vi "Test Sequence Constructor.vi"() -> ()   [LabVIEW 2014]
panel:
  in  "Sequence 2":string(tree)
  out "Steps":string[](array[string])
  out "Values":string[](array[string])
  in  "add":bool
  in  "Steps":string(tree)
  in  "Sequence":string(tree)
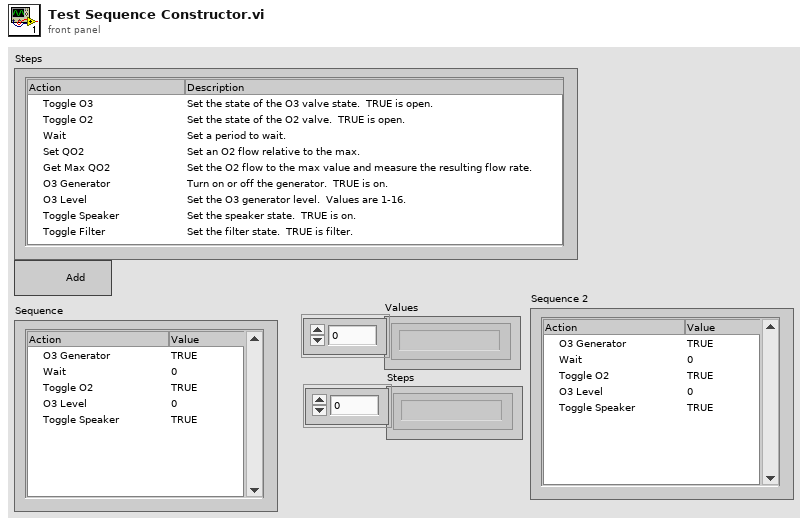
[diagram p1: front panel]
types:
  T1 = typedef "eventvkey.ctl" = enum16{"ASCII", "Enter", "Return", "Shift", "Ctrl", "Alt", "Cmd", "Opt", "Caps", "NumLock", "Clear", "Break", "Up", "Down", "Left", "Right", "Insert", "Delete", "Home", "End", "PageUp", "PageDown", "Escape", "Help", "Pause", "ScrollLock", "F1", "F2", "F3", "F4", "F5", "F6", "F7", "F8", "F9", "F10", "F11", "F12", "F13", "F14", "F15", "F16", "F17", "F18", "F19", "F20", "F21", "F22", "F23", "F24", "Play", "VolumeUp", "VolumeDown", "Mute", "Two Byte Char"}
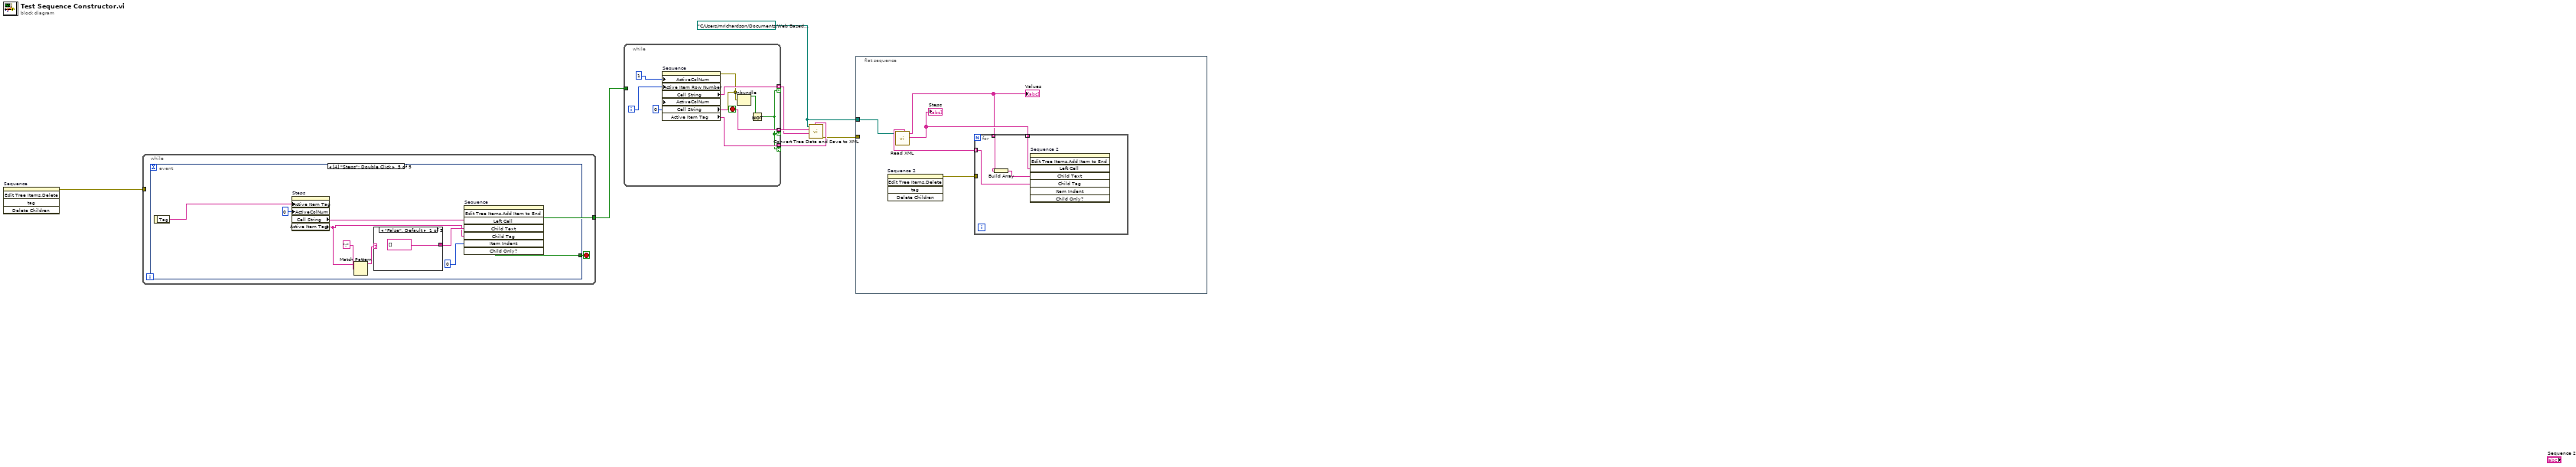
[diagram p0: block diagram]
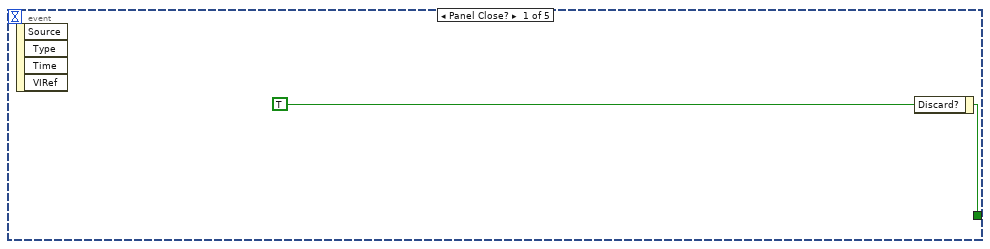
[diagram p2: hidden frame]
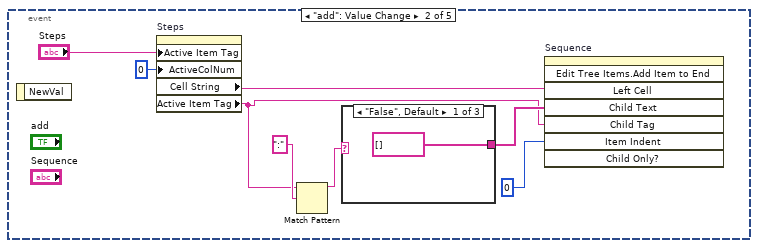
[diagram p3: hidden frame]
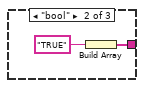
[diagram p4: hidden frame]
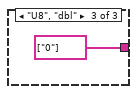
[diagram p5: hidden frame]
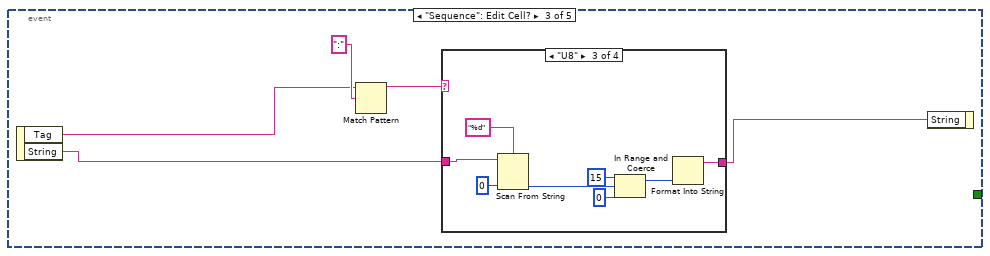
[diagram p6: hidden frame]
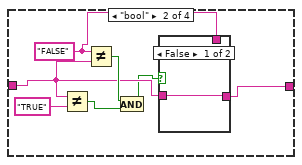
[diagram p8: hidden frame]
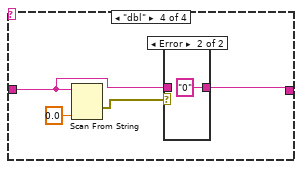
[diagram p10: hidden frame]
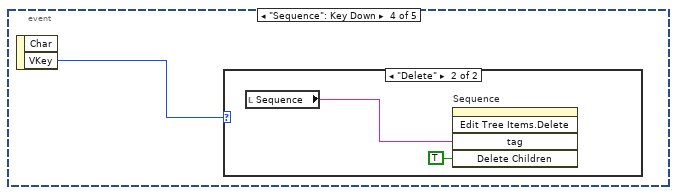
[diagram p12: hidden frame]
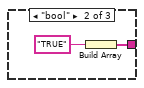
[diagram p14: hidden frame]
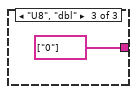
[diagram p15: hidden frame]
diagram:
  w1 = path "C:/Users/mrichardson/Documents/Web Based Version Control SW/Instruments/cPAS/Test/test.xml" ("file")
  n1 = invoke on="Sequence" class="Tree (strict)" method="Edit Tree Items.Delete"() -> (error out=w7:errorcluster)  [unwired: 5 in, 4 out]
  n2 = while {
    tunnel: w7 -> [_]
    tunnel: [w8] -> w6
    stop <- w8 stop-if-true
    n3 = event shown="[4] \"Steps\": Double Click" {
      selector: _ -> [_ _ _ _ _]
      dyn-events: _ -> [_ _ _ _ _]
      timeout: _ -> [_ _ _ _ _]
      tunnel: [w9 _ _ _ _] -> w8
      event Panel Close? {
        w9 = TRUE ("Discard?")
        n4 = event-data() -> ()  [unwired: 1 in, 4 out]
        n5 = event-data("Discard?"=w9) -> ()  [unwired: 1 in, 1 out]
      }
      event "add": Value Change {
        n6 = event-data() -> ()  [unwired: 1 in, 1 out]
        n7 = property on="Steps" class="Tree (strict)"("Active Item Tag"="Steps", "ActiveColNum"=0 ("Active Cell:Active Column Number")) -> ("Cell String"=w15:string, "Active Item Tag"=w10:string)  [unwired: 2 in, 2 out]
        n8 = Match Pattern(string=w10, regular expression=":" ("search string/char (-)")) -> (before substring=w11:string)  [unwired: 1 in, 3 out]
        n9 = case shown="\"False\", Default" w11 {
          tunnel: [string[] [] w19 string[] ["0"]] -> w13
          frame "False", Default {
          }
          frame "bool" {
            n10 = Build Array("TRUE") -> (w19:string[])
          }
          frame "U8", "dbl" {
          }
        }
        n11 = invoke on="Sequence" class="Tree (strict)" method="Edit Tree Items.Add Item to End"("Left Cell"=w15, "Child Text"=w13, "Child Tag"=w10, "Item Indent"=0 ("New Item Indentation")) -> ()  [unwired: 4 in, 8 out]
      }
      event "Sequence": Edit Cell? {
        n12 = event-data() -> ("Tag"=w22:string, "String"=w24:string)  [unwired: 1 in]
        n13 = Match Pattern(string=w22, regular expression=":" ("search string/char (-)")) -> (before substring=w25:string)  [unwired: 1 in, 3 out]
        n14 = case shown="\"U8\"" w25 {
          tunnel: w24 -> [w27 w31 w44 w46]
          tunnel: [w27 w28 w37 w45] -> w23
          frame "False", Default {
          }
          frame "bool" {
            w29 = "FALSE" ("x")
            n15 = Not Equal?(x=w31, y="TRUE") -> (x != y?=w33:bool)
            n16 = Not Equal?(x=w29, y=w31) -> (x != y?=w32:bool)
            n17 = And(x=w32, y=w33) -> (x .and. y?=w30:bool)
            n18 = case shown="False" w30 {
              tunnel: w31 -> [w35 _]
              tunnel: [w35 w36] -> w28
              tunnel: w29 -> [_ w36]
              frame False {
              }
              frame True {
              }
            }
          }
          frame "U8" {
            n19 = Scan From String(format string="%d", input string=w44, default 1=u8 0 ("default value 1")) -> (output 1=w41:u8)  [unwired: 2 in, 3 out]
            n20 = In Range and Coerce(upper limit=u8 15, x=w41, lower limit=u8 0) -> (coerced(x)=w38:u8)  [unwired: 1 out]
            n21 = Format Into String(w38) -> (resulting string=w37:string)  [unwired: 3 in, 1 out]
          }
          frame "dbl" {
            n22 = Scan From String(input string=w46, default 1=0.0 ("default value 1")) -> (error out=w47:errorcluster)  [unwired: 4 in, 2 out]
            n23 = case shown="Error" w47 {
              tunnel: w46 -> [w49 _]
              tunnel: [w49 "0" ("NewVal")] -> w45
              frame No Error {
              }
              frame Error {
              }
            }
          }
        }
        n24 = event-data("String"=w23) -> ()  [unwired: 1 in, 1 out]
      }
      event "Sequence": Key Down {
        n25 = event-data() -> ("VKey"=w51:T1)  [unwired: 1 in, 1 out]
        n26 = case shown="\"Delete\"" w51 {
          frame "ASCII", Default {
          }
          frame "Delete" {
            n27 = local read "Sequence"() -> (w53:string)
            n28 = invoke on="Sequence" class="Tree (strict)" method="Edit Tree Items.Delete"("tag"=w53, "Delete Children"=TRUE ("Delete Children?")) -> ()  [unwired: 3 in, 5 out]
          }
        }
      }
      event "Steps": Double Click {
        n29 = event-data() -> ("Tag"=w54:string)  [unwired: 1 in]
        n30 = property on="Steps" class="Tree (strict)"("Active Item Tag"=w54, "ActiveColNum"=0 ("Active Cell:Active Column Number")) -> ("Cell String"=w60:string, "Active Item Tag"=w55:string)  [unwired: 2 in, 2 out]
        n31 = Match Pattern(string=w55, regular expression=":" ("search string/char (-)")) -> (before substring=w56:string)  [unwired: 1 in, 3 out]
        n32 = case shown="\"False\", Default" w56 {
          tunnel: [string[] [] w63 string[] ["0"]] -> w58
          frame "False", Default {
          }
          frame "bool" {
            n33 = Build Array("TRUE") -> (w63:string[])
          }
          frame "U8", "dbl" {
          }
        }
        n34 = invoke on="Sequence" class="Tree (strict)" method="Edit Tree Items.Add Item to End"("Left Cell"=w60, "Child Text"=w58, "Child Tag"=w55, "Item Indent"=0 ("New Item Indentation")) -> ()  [unwired: 4 in, 8 out]
      }
    }
  }
  n35 = while {
    tunnel: [w72] -> w4 mode=indexing if=w66
    tunnel: w6 -> [_]
    tunnel: [w68] -> w5 mode=indexing if=w66
    tunnel: [w67] -> w3 mode=indexing if=w66
    i -> [w73]
    stop <- w70 stop-if-true
    n36 = property on="Sequence" class="Tree (strict)"("ActiveColNum"=1 ("Active Cell:Active Column Number"), "Active Item Row Number"=w73, "ActiveColNum"=0 ("Active Cell:Active Column Number")) -> (error out=w70:errorcluster, "Cell String"=w72:string, "Cell String"=w68:string, "Active Item Tag"=w67:string)  [unwired: 2 in, 1 out]
    n37 = Unbundle(w70) -> ("status"=w71:bool)  [unwired: 2 out]
    n38 = Not(x=w71) -> (.not. x?=w66:bool)
  }
  n39 = call "Convert Tree Data and Save to XML.vi"("tag"=w3, "Value"=w4, "Step"=w5, "file"=w1) -> ("error out"=w2:errorcluster)  [unwired: 5 in, 2 out]
  n40 = flat-sequence {
    tunnel: w2 -> [_]
    tunnel: w1 -> [w75]
    frame #0 {
      n41 = invoke on="Sequence 2" class="Tree (strict)" method="Edit Tree Items.Delete"() -> (error out=w79:errorcluster)  [unwired: 5 in, 4 out]
      n42 = call "Read XML.vi"("path"=w75) -> ("Steps"=w77:string[], "Values"=w76:string[], "tags"=w78:string[])  [unwired: 6 in, 2 out]
      "Values" <- w76
      "Steps" <- w77
      n43 = for {
        tunnel: w79 -> [_]
        tunnel: w78 -> [w83] mode=indexing
        tunnel: w77 -> [w82] mode=indexing
        tunnel: w76 -> [w81] mode=indexing
        n44 = Build Array(w81) -> (w80:string[])
        n45 = invoke on="Sequence 2" class="Tree (strict)" method="Edit Tree Items.Add Item to End"("Left Cell"=w82, "Child Text"=w80, "Child Tag"=w83) -> ()  [unwired: 5 in, 8 out]
      }
    }
  }
